vi "backup_data_on_network.vi"(11 "Filepath in":path) -> (3 "Filepath out":path)   [LabVIEW 2018]
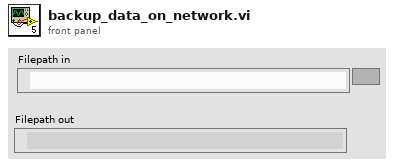
[diagram p1: front panel]
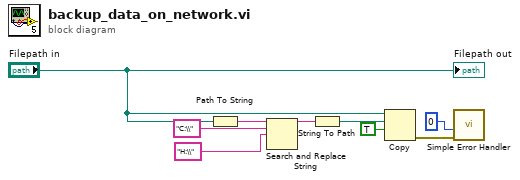
[diagram p0: block diagram]
diagram:
  n1 = Path To String(path="Filepath in") -> (string=w5:string)
  n2 = Search and Replace String(input string=w5, search string="C:\\", replace string="H:\\") -> (result string=w7:string)  [unwired: 5 in, 3 out]
  n3 = String To Path(string=w7) -> (path=w6:path)
  n4 = Copy(9:TRUE ("overwrite (F)"), 10:w6, 11:"Filepath in") -> (0:w9:errorcluster)  [unwired: 2 in, 2 out]
  n5 = call <vilib>:"Simple Error Handler.vi"("type of dialog (OK msg:1)"=0, "error in (no error)"=w9) -> ()  [unwired: 3 in, 5 out]
  "Filepath out" <- "Filepath in"
